vi "Go to Ready.vi"(8 "error in (no error)":errorcluster, 11 "Ready in":refnum<class "Ready.lvclass">) -> (0 "error out":errorcluster, 3 "Process State out":refnum<class "State Actor.lvclass">)   [LabVIEW 2014, in "States.lvlib" / "Ready.lvclass"]
doc: "This override disables entry behavior when entering the Idle state."
uses:
  Ready.lvclass
  <vilib>/NI/Actors/State Actor/State Actor/State Actor.lvclass
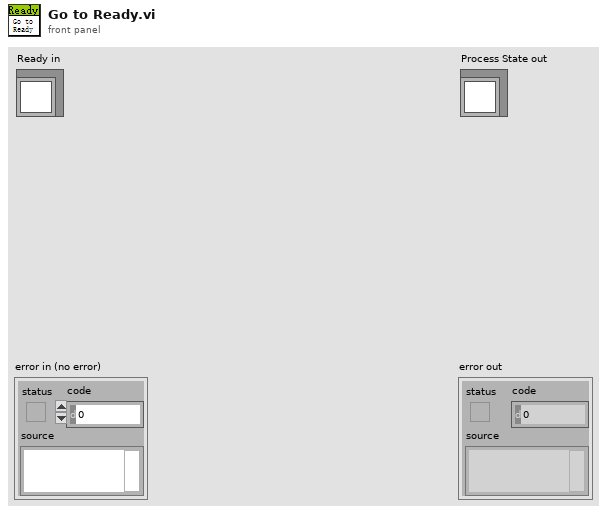
[diagram p1: front panel]
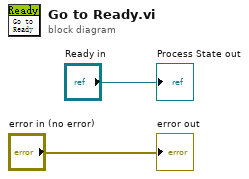
[diagram p0: block diagram]
diagram:
  "error out" <- "error in (no error)"
  "Process State out" <- "Ready in"
